vi "SearchClassCode.vi"(8 "error in (no error)":errorcluster, 11 "CS in":refnum<class "CS.lvclass">) -> (0 "error out":errorcluster, 3 "CS out":refnum<class "CS.lvclass">)   [LabVIEW 2013, in "CS.lvclass"]
uses:
  CS.lvclass
  baseClass/baseClass.lvclass
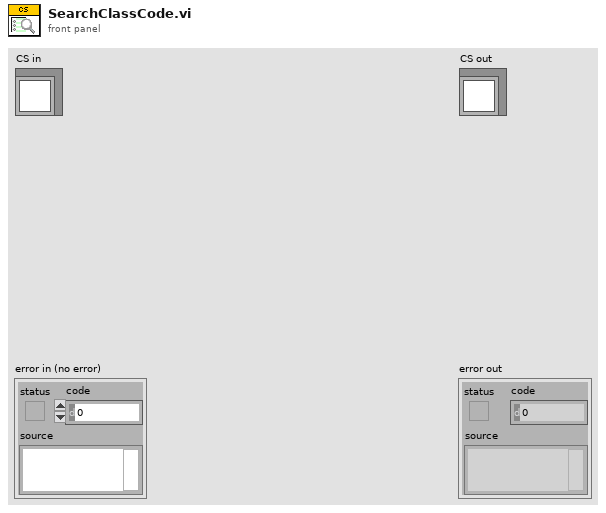
[diagram p1: front panel]
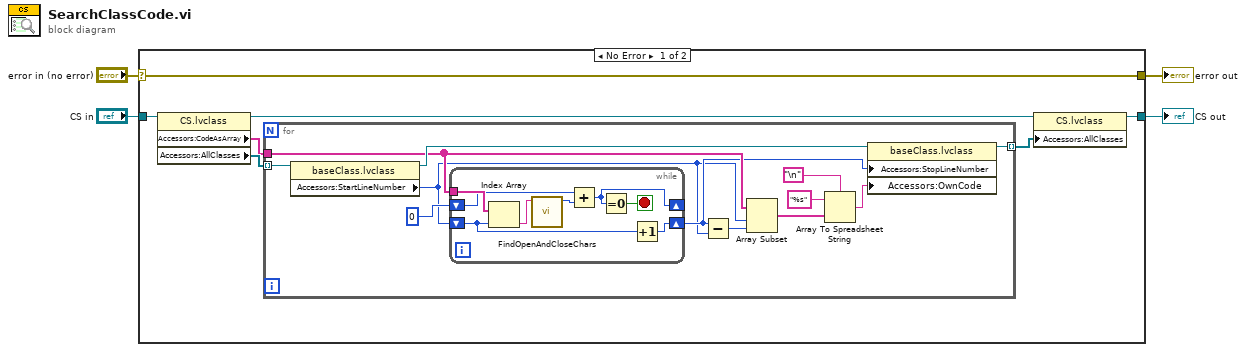
[diagram p0: block diagram]
diagram:
  n1 = case shown="No Error" "error in (no error)" {
    selector: "error in (no error)" -> [w10 w33]
    tunnel: [w10 w33] -> w3
    tunnel: [w6 w32] -> w1
    tunnel: "CS in" -> [w11 w32]
    frame No Error {
      n2 = property class="CS.lvclass"(reference=w11) -> (reference out=w9:refnum<class "CS.lvclass">, "Accessors:CodeAsArray"=w7:string[], "Accessors:AllClasses"=w8:refnum<class "baseClass.lvclass">[])  [unwired: 1 in, 1 out]
      n3 = for {
        tunnel: w8 -> [w23] mode=indexing
        tunnel: w7 -> [w20]
        tunnel: [w12] -> w5 mode=indexing
        n4 = property class="baseClass.lvclass"(reference=w23) -> (reference out=w21:refnum<class "baseClass.lvclass">, "Accessors:StartLineNumber"=w18:u32)  [unwired: 1 in, 1 out]
        n5 = while {
          shift-right: [w25] -> w19
          shift-left: w18 -> [w24]
          shift-right: [w28] -> _
          shift-left: 0 -> [w30]
          tunnel: w20 -> [w31]
          stop <- w27 stop-if-true
          n6 = Index Array(array=w31, index=w24) -> (element=w26:string)
          n7 = call "FindOpenAndCloseChars.vi"("String"=w26) -> ("Counter"=w29:i32)  [unwired: 7 in, 3 out]
          n8 = Add(x=w30, y=w29) -> (x+y=w28:i32)
          n9 = Equal To 0?(x=w28) -> (x = 0?=w27:bool)
          n10 = Increment(x=w24) -> (x+1=w25:u32)
        }
        n11 = Subtract(x=w19, y=w18) -> (x-y=w17:u32)
        n12 = Array Subset(array=w20, index=w18, length=w17) -> (w16:string[])
        n13 = Array To Spreadsheet String(delimiter (Tab)="\n", array=w16, 3:"%s" ("format string")) -> (spreadsheet string=w13:string)
        n14 = property class="baseClass.lvclass"(reference=w21, "Accessors:StopLineNumber"=w19, "Accessors:OwnCode"=w13) -> (reference out=w12:refnum<class "baseClass.lvclass">)  [unwired: 1 in, 1 out]
      }
      n15 = property class="CS.lvclass"(reference=w9, "Accessors:AllClasses"=w5) -> (reference out=w6:refnum<class "CS.lvclass">)  [unwired: 1 in, 1 out]
    }
    frame Error {
    }
  }
  "error out" <- w3
  "CS out" <- w1
